vi "Status.vi"(8 "error in (no error)":errorcluster, 10 "Internal?":bool, 11 "Lauda Settings":T1) -> (0 "error out":errorcluster, 1 "Connection Error":bool, 2 "Running":bool, 3 "Lauda Settings":T1, 4 "Temp":dbl, 5 "No external Sensor":bool, 6 "Pump Speed":i32)   [LabVIEW 2018, in "Lauda TCU.lvlib"]
uses:
  Lauda TCU.lvlib
  Lauda Settings.ctl
  <vilib>/Utility/error.llb/DialogType.ctl
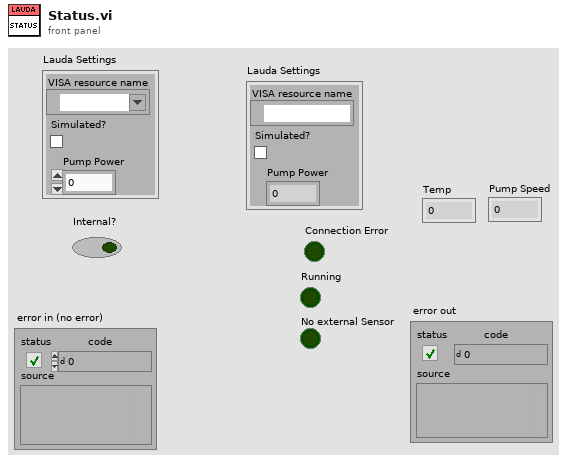
[diagram p1: front panel]
types:
  T1 = typedef "Lauda TCU.lvlib/Lauda Settings.ctl" = cluster{"VISA resource name":refnum<visa-resource-name>, "Simulated?":bool, "Pump Power":i32}
  T2 = typedef "DialogType.ctl" = u16
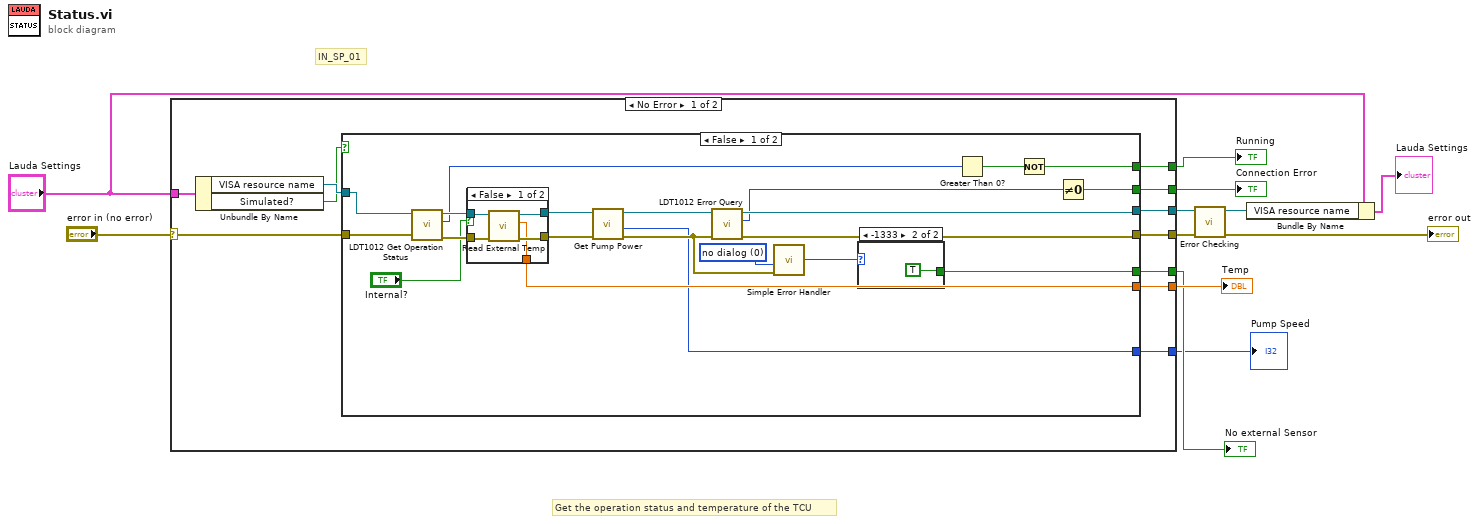
[diagram p0: block diagram]
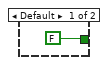
[diagram p2: hidden frame]
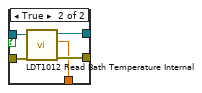
[diagram p3: hidden frame]
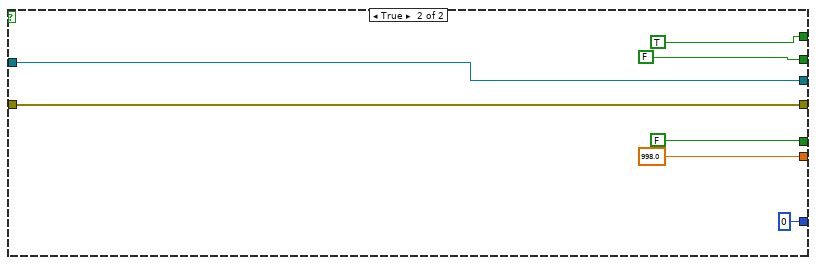
[diagram p4: hidden frame]
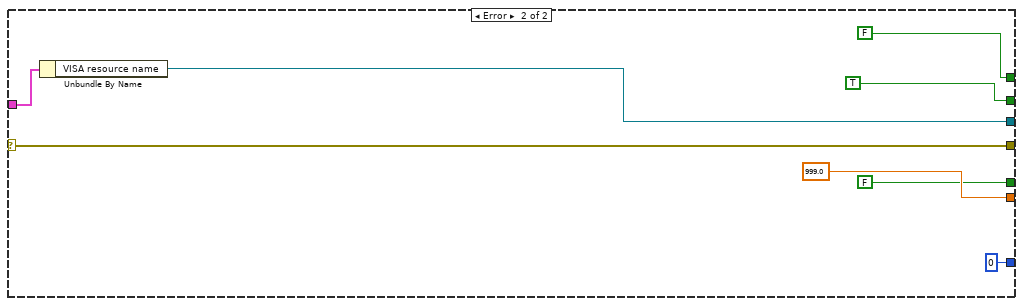
[diagram p5: hidden frame]
diagram:
  # "IN_SP_01"
  # "Get the operation status and temperature of the TCU"
  n1 = case shown="No Error" "error in (no error)" {
    selector: "error in (no error)" -> [w23 w71]
    tunnel: "Lauda Settings" -> [w21 w70]
    tunnel: [w22 w71] -> w10
    tunnel: [w19 w69] -> w11
    tunnel: [w17 TRUE] -> w5
    tunnel: [w16 FALSE] -> w4
    tunnel: [w15 999.0 ("Internal Bath Temperature")] -> w3
    tunnel: [w14 FALSE] -> w2
    tunnel: [w13 0 ("Pump Speed")] -> w1
    frame No Error {
      n2 = Unbundle By Name(w21) -> ("VISA resource name"=w20:refnum<visa-resource-name>, "Simulated?"=w18:bool)
      n3 = case shown="False" w18 {
        tunnel: w23 -> [w43 w63]
        tunnel: [w38 w63] -> w22
        tunnel: [w39 w62] -> w19
        tunnel: w20 -> [w44 w62]
        tunnel: [w36 FALSE] -> w17
        tunnel: [w24 TRUE] -> w16
        tunnel: [w35 998.0 ("Internal Bath Temperature")] -> w15
        tunnel: [w32 FALSE] -> w14
        tunnel: [w26 0 ("Pump Speed")] -> w13
        frame False {
          w31 = T2 0 items=["no dialog", "OK message", "continue or stop message", "OK message + warnings", "continue/stop + warnings"] ("type of dialog (OK msg:1)")
          n4 = call "LDT1012 Get Operation Status.vi"("error in (no error)"=w43, "VISA session"=w44) -> ("error out"=w41:errorcluster, "Get Operation Status"=w40:u8, "dup VISA session"=w42:refnum<visa-resource-name>)  [unwired: 7 in]
          n5 = case shown="False" "Internal?" {
            tunnel: w42 -> [w50 w56]
            tunnel: w41 -> [w49 w55]
            tunnel: [w51 w54] -> w30
            tunnel: [w48 w53] -> w28
            tunnel: [w47 w52] -> w35
            frame False {
              n6 = call "Read External Temp.vi"("error in (no error)"=w49, "VISA session"=w50) -> ("error out"=w48:errorcluster, "External PT100 Temperature"=w47:dbl, "dup VISA session"=w51:refnum<visa-resource-name>)  [unwired: 7 in]
            }
            frame True {
              n7 = call "LDT1012 Read Bath Temperature Internal.vi"("error in (no error)"=w55, "VISA session"=w56) -> ("error out"=w53:errorcluster, "Internal Bath Temperature"=w52:dbl, "dup VISA session"=w54:refnum<visa-resource-name>)  [unwired: 7 in]
            }
          }
          n8 = call "Get Pump Power.vi"("error in (no error)"=w28, "VISA session"=w30) -> ("error out"=w27:errorcluster, "Pump Speed"=w26:i32, "dup VISA session"=w29:refnum<visa-resource-name>)  [unwired: 6 in, 1 out]
          n9 = call "LDT1012 Error Query.vi"("error in (no error)"=w27, "VISA session"=w29) -> ("error out"=w38:errorcluster, "Error"=w37:u8, "dup VISA session"=w39:refnum<visa-resource-name>)  [unwired: 5 in, 2 out]
          n10 = call <vilib>:"Simple Error Handler.vi"("type of dialog (OK msg:1)"=w31, "error in (no error)"=w27) -> ("code out"=w33:i32)  [unwired: 3 in, 4 out]
          n11 = case shown="-1333" w33 {
            tunnel: [FALSE TRUE] -> w32
            frame Default {
            }
            frame -1333 {
            }
          }
          n12 = Greater Than 0?(x=w40) -> (x > 0?=w25:bool)
          n13 = Not(x=w25) -> (.not. x?=w24:bool)
          n14 = Not Equal To 0?(x=w37) -> (x != 0?=w36:bool)
        }
        frame True {
        }
      }
    }
    frame Error {
      n15 = Unbundle By Name(w70) -> ("VISA resource name"=w69:refnum<visa-resource-name>)
    }
  }
  "Connection Error" <- w5
  "Running" <- w4
  "Temp" <- w3
  "No external Sensor" <- w2
  "Pump Speed" <- w1
  n16 = call "Error Checking.vi"("error in (no error)"=w10, "VISA resource name"=w11) -> ("error out"=→"error out":errorcluster, "VISA resource name"=w8:refnum<visa-resource-name>)  [unwired: 7 in, 1 out]
  n17 = Bundle By Name(cluster="Lauda Settings", "VISA resource name"=w8) -> (→"Lauda Settings":T1)
